vi "getAttributeByName.vi"(8 "error in (no error)":errorcluster, 10 "name":string, 11 "NativeXML in":refnum<class "NativeXML.lvclass">) -> (0 "error out":errorcluster, 2 "Attribute String":string, 3 "NativeXML out":refnum<class "NativeXML.lvclass">)   [LabVIEW 2011, in "Tools.lvlib" / "xml.lvlib" / "NativeXML.lvclass"]
uses:
  NativeXML.lvclass
  NativeXML.lvclass/NativeXML.ctl
  <vilib>/xml/Close Reference(Node).vi
  <vilib>/xml/Close Reference(NNMap).vi
  Program Files/National Instruments/LabVIEW 2011/resource/objmgr/DOMUserDefRef.rc
  <vilib>/xml/NI_XML.lvlib
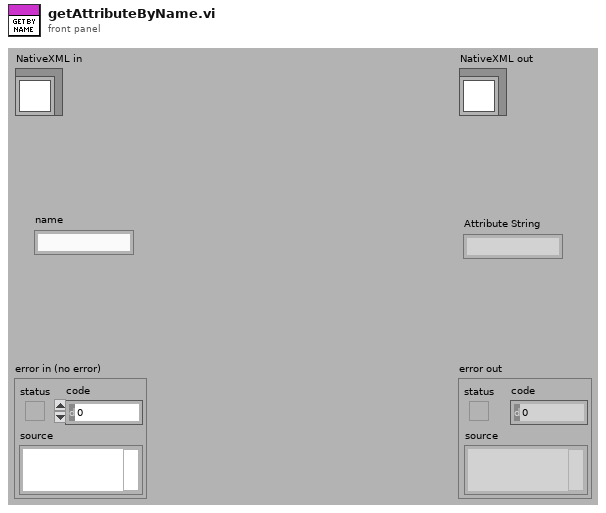
[diagram p1: front panel]
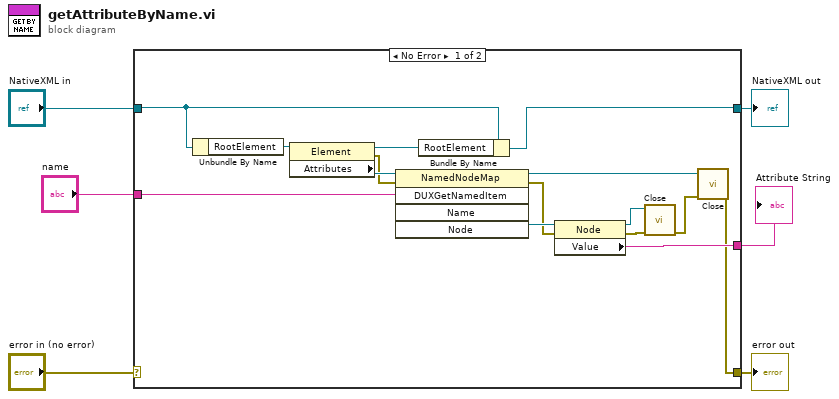
[diagram p0: block diagram]
diagram:
  n1 = case shown="No Error" "error in (no error)" {
    selector: "error in (no error)" -> [_ w23]
    tunnel: [w12 w23] -> w5
    tunnel: [w7 w22] -> w3
    tunnel: "NativeXML in" -> [w8 w22]
    tunnel: "name" -> [w19 _]
    tunnel: [w17 _] -> w1
    frame No Error {
      n2 = Unbundle By Name(w8) -> ("RootElement"=w21:refnum<k20>)
      n3 = property class="Element"(reference=w21) -> (reference out=w9:refnum<k20>, error out=w10:errorcluster, "Attributes"=w20:refnum<k20>)  [unwired: 1 in]
      n4 = invoke class="NamedNodeMap" method="DUXGetNamedItem"(reference=w20, error in=w10, "Name"=w19) -> (reference out=w14:refnum<k20>, error out=w11:errorcluster, "Node"=w18:refnum<k20>)  [unwired: 2 in, 2 out]
      n5 = Bundle By Name(cluster=w8, "RootElement"=w9) -> (w7:refnum<class "NativeXML.lvclass">)
      n6 = property class="Node"(reference=w18, error in=w11) -> (reference out=w16:refnum<k20>, error out=w15:errorcluster, "Value"=w17:string)
      n7 = call-poly <vilib>:"Close.vi"("error in (no error)"=w15, "node"=w16) -> ("error out"=w13:errorcluster)  [unwired: 7 in]
      n8 = call-poly <vilib>:"Close.vi"("error in (no error)"=w13, "named node map"=w14) -> ("error out"=w12:errorcluster)  [unwired: 7 in]
    }
    frame Error {
    }
  }
  "error out" <- w5
  "NativeXML out" <- w3
  "Attribute String" <- w1
